vi "save_image(SubVI).vi"(7 "file name":string, 8 "error in (no error)":errorcluster, 9 "Image Type":T1 items=["Grayscale (U8)", "Grayscale (I16)", "Grayscale (SGL)", "Complex (CSG)", "RGB (U32)", "HSL (U32)", "RGB (U64)", "Grayscale (U16)"], 10 "Image":T2, 11 "base path":path) -> (0 "error out":errorcluster, 3 "Image Out (duplicate)":T2)   [LabVIEW 2020]
doc: "salva un immagine in memoria.\nrichiede in ingresso l'immagine da salvare (Image)."
uses:
  <vilib>/vision/Image Controls.llb/IMAQ Image.ctl
panel:
  in  "stop":bool
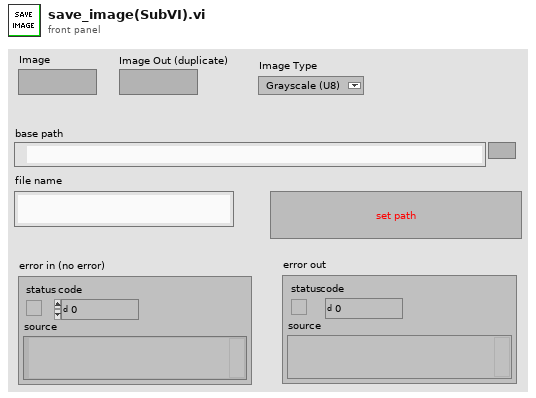
[diagram p1: front panel]
types:
  T1 = typedef "Image Type" = u32
  T2 = typedef "IMAQ Image.ctl" = refnum<image>
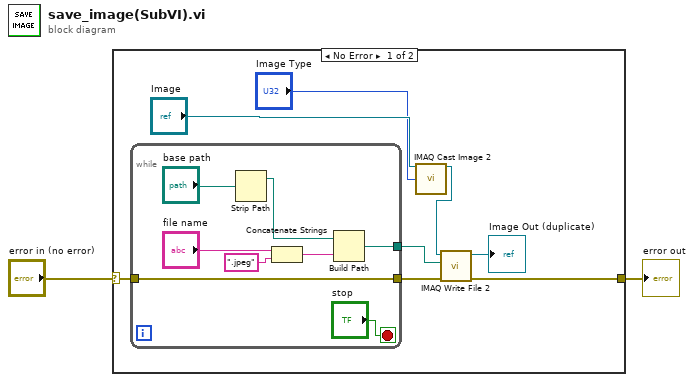
[diagram p0: block diagram]
diagram:
  n1 = case shown="No Error" "error in (no error)" {
    selector: "error in (no error)" -> [w7 w19]
    tunnel: [w10 w19] -> w2
    frame No Error {
      n2 = while {
        tunnel: [w16] -> w9
        tunnel: w7 -> [w18]
        tunnel: [w18] -> w6
        stop <- "stop" stop-if-true
        n3 = Strip Path(path="base path") -> (stripped path=w11:path)  [unwired: 1 out]
        n4 = Concatenate Strings("file name", ".jpeg" ("string")) -> (w14:string)
        n5 = Build Path(base path=w11, name or relative path=w14) -> (appended path=w16:path)
      }
      n6 = call "IMAQ Cast Image 2"("Image Src"="Image", "Image Type"="Image Type") -> ("Image Dst Out"=w4:T2)  [unwired: 12 in, 1 out]
      n7 = call-poly "IMAQ Write File 2"("error in (no error)"=w6, "File Path"=w9, "Image"=w4) -> ("error out"=w10:errorcluster, "Image Out (duplicate)"=→"Image Out (duplicate)":T2)  [unwired: 7 in]
    }
    frame Error {
    }
  }
  "error out" <- w2
